vi "aft_LMS_Edit_VIs.vi"(6 "read coefficient? (F)":bool, 8 "error in":errorcluster {"code" min=0 max=0}, 9 "filter name":string, 10 "fixed-point LMS settings":T1 {"fixed-point configurations"."step size integer word length" min=0 max=0; "fixed-point configurations"."step size word length" min=0 max=0; "fixed-point configurations"."w(n) integer word length" min=0 max=0; "fixed-point configurations"."w(n) word length" min=0 max=0; "fixed-point configurations"."d(n) integer word length" min=0 max=0; "fixed-point configurations"."d(n) word length" min=0 max=0; "fixed-point configurations"."x(n) integer word length" min=0 max=0; "fixed-point configurations"."x(n) word length" min=0 max=0; "step size" min=0.0 max=0.0; "filter length" min=0 max=0}, 11 "VI ref":refnum<vi>) -> (0 "error out":errorcluster {"code" min=0 max=0})   [LabVIEW 2017, in "NI_AdaptiveFilter.lvlib"]
uses:
  <vilib>/addons/Adaptive Filters/NI_AdaptiveFilter.lvlib
  <vilib>/fxp/LVFixedPointOverflowPolicyTypeDef.ctl
  <vilib>/fxp/LVFixedPointQuantizationPolicyTypeDef.ctl
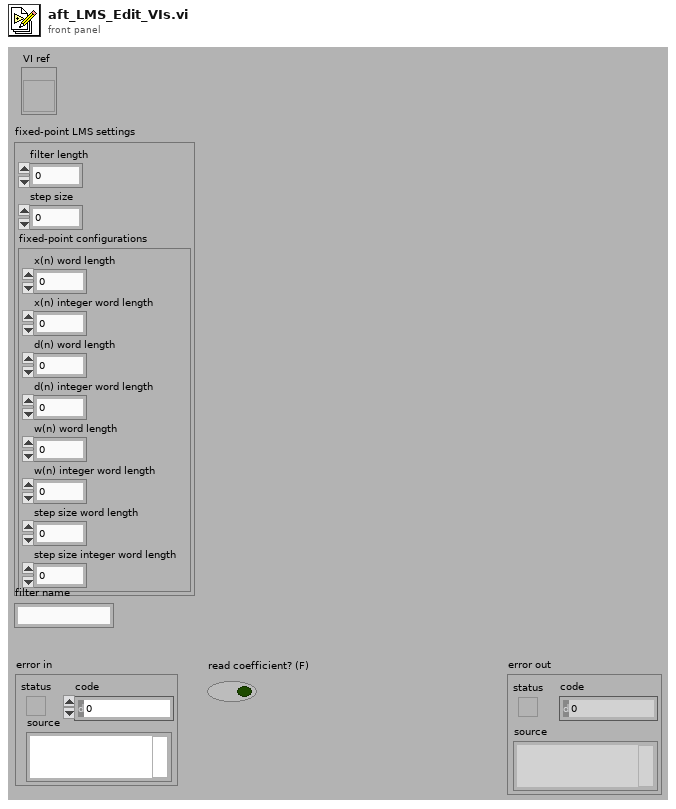
[diagram p1: front panel]
types:
  T1 = cluster{"filter length":i32, "step size":dbl, "fixed-point configurations":cluster{"x(n) word length":i32, "x(n) integer word length":i32, "d(n) word length":i32, "d(n) integer word length":i32, "w(n) word length":i32, "w(n) integer word length":i32, "step size word length":i32, "step size integer word length":i32}}
  T2 = typedef "LVFixedPointOverflowPolicyTypeDef.ctl" = enum32{"Wrap", "Saturate"}
  T3 = cluster{"x(n) word length":i32, "x(n) integer word length":i32, "d(n) word length":i32, "d(n) integer word length":i32, "w(n) word length":i32, "w(n) integer word length":i32, "step size word length":i32, "step size integer word length":i32}
  T4 = cluster{bool, u32, "x(n) integer word length":i32}
  T5 = cluster{bool, u32, "d(n) integer word length":i32}
  T6 = cluster{bool, u32, "step size integer word length":i32}
  T7 = typedef "LVFixedPointRepBitsTypeDef.ctl" = cluster{"Signed":bool, "Word Length":u32, "Integer Word Length":i32}
  T8 = typedef "LVFixedPointQuantizationPolicyTypeDef.ctl" = enum32{"Truncate", "Round-Half-Up (Asymmetric)", "Round-Half-Even"}
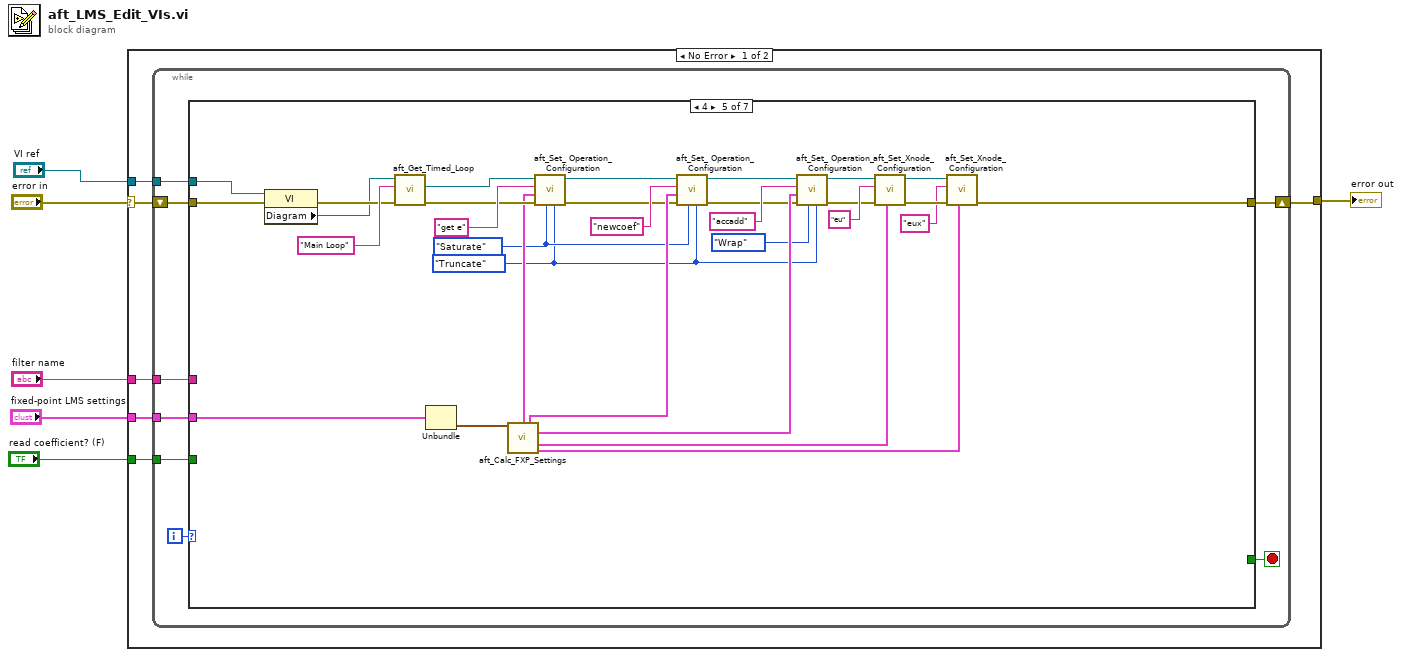
[diagram p0: block diagram]
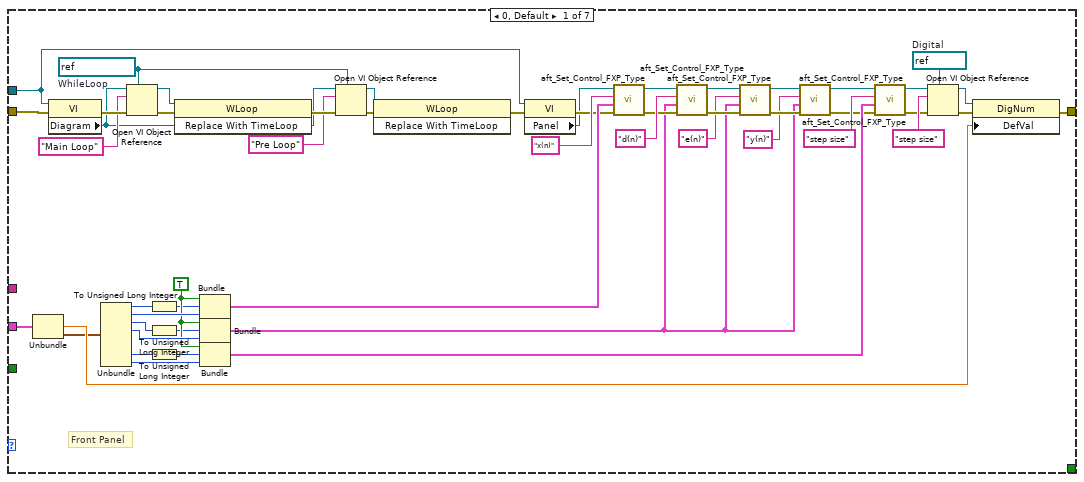
[diagram p2: hidden frame]
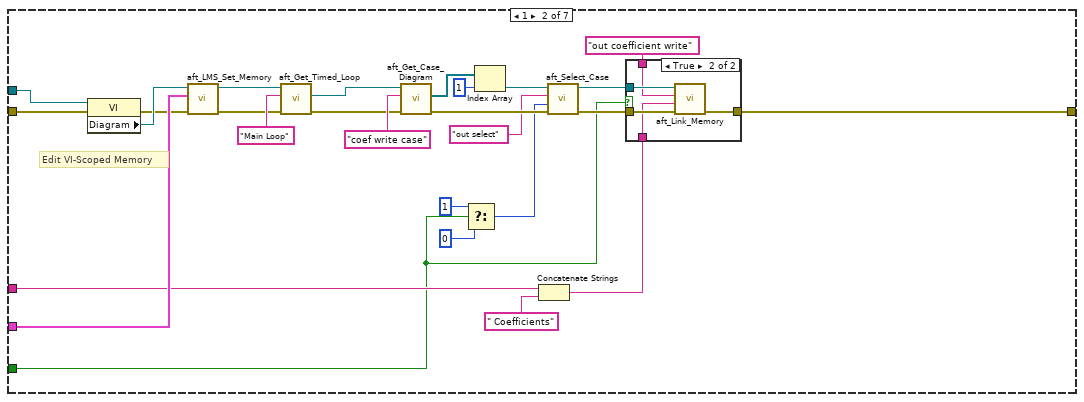
[diagram p3: hidden frame]
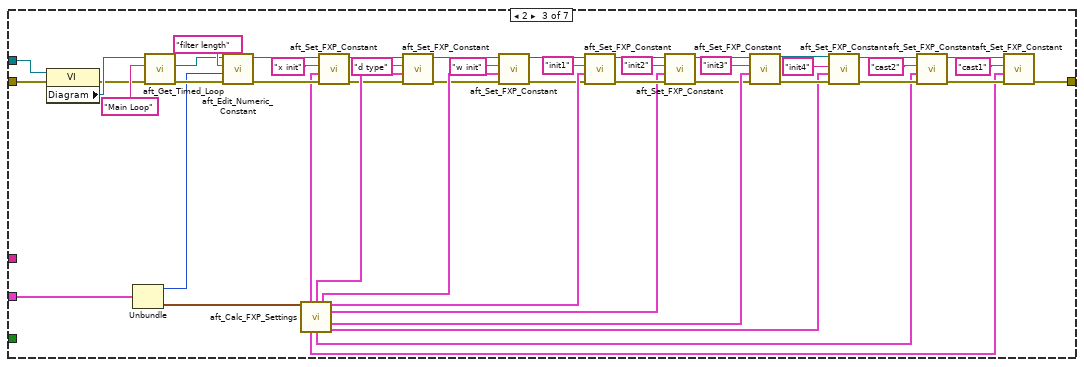
[diagram p5: hidden frame]
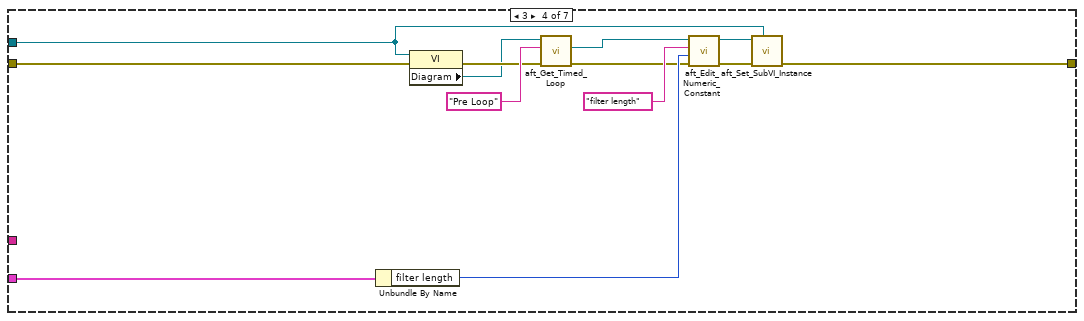
[diagram p6: hidden frame]
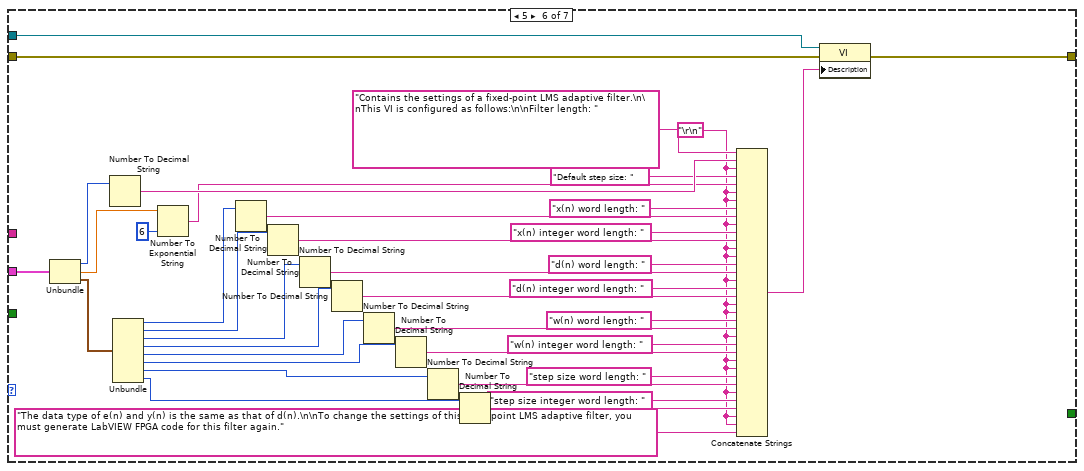
[diagram p7: hidden frame]
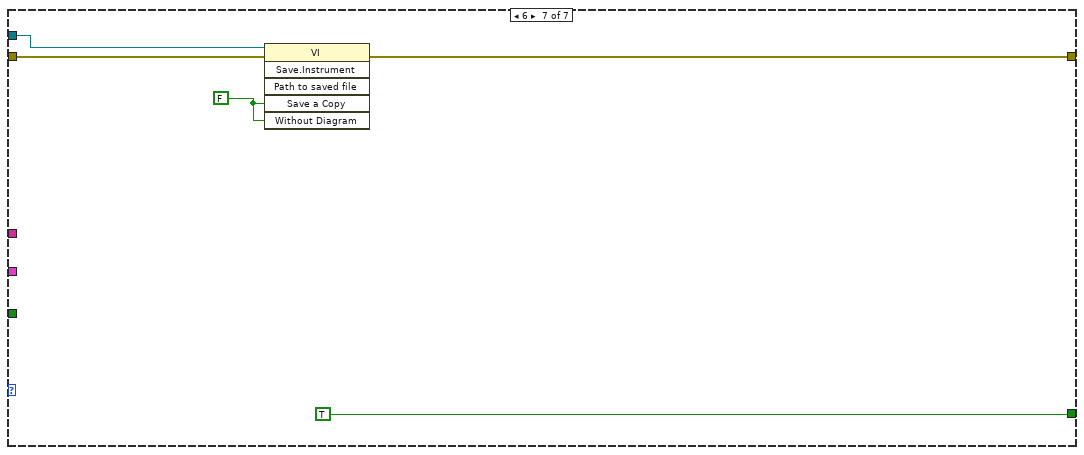
[diagram p8: hidden frame]
diagram:
  n1 = case shown="No Error" "error in" {
    selector: "error in" -> [w10 w241]
    tunnel: "VI ref" -> [w12 _]
    tunnel: [w9 w241] -> w6
    tunnel: "fixed-point LMS settings" -> [w11 _]
    tunnel: "filter name" -> [w8 _]
    tunnel: "read coefficient? (F)" -> [w7 _]
    frame No Error {
      n2 = while {
        tunnel: w12 -> [w20]
        tunnel: w11 -> [w19]
        shift-right: [w17] -> w9
        shift-left: w10 -> [w18]
        tunnel: w8 -> [w15]
        tunnel: w7 -> [w13]
        i -> [w16]
        stop <- w14 stop-if-true
        n3 = case shown="4" w16 {
          tunnel: w20 -> [w33 w94 w140 w154 w187 w197 w237]
          tunnel: w19 -> [w43 w96 w143 w161 w192 w233 _]
          tunnel: w18 -> [w34 w98 w148 w164 w196 w235 w239]
          tunnel: [w21 w78 w107 w153 w173 w234 w238] -> w17
          tunnel: w15 -> [_ w79 _ _ _ _ _]
          tunnel: [_ _ _ _ _ _ TRUE] -> w14
          tunnel: w13 -> [_ w77 _ _ _ _ _]
          frame 0, Default {
            w28 = refnum<vi> refnum  # WhileLoop
            w61 = refnum<vi> refnum  # Digital
            w58 = TRUE
            # "Front Panel"
            n4 = Unbundle(w43) -> ("step size"=w64:dbl, "fixed-point configurations"=w35:T3)  [unwired: 1 out]
            n5 = property class="VI"(reference=w33, error in=w34) -> (error out=w32:errorcluster, "Diagram"=w26:refnum<vi>)  [unwired: 1 out]
            n6 = Unbundle(w35) -> ("x(n) word length"=w66:i32, "x(n) integer word length"=w67:i32, "d(n) word length"=w68:i32, "d(n) integer word length"=w69:i32, "step size word length"=w70:i32, "step size integer word length"=w71:i32)  [unwired: 2 out]
            n7 = Open VI Object Reference(7:w28, 8:w32, 10:"Main Loop" ("name/order"), 11:w26) -> (0:w30:errorcluster, 3:w29:refnum<vi>)
            n8 = To Unsigned Long Integer(number=w66) -> (unsigned 32bit integer=w51:u32)
            n9 = To Unsigned Long Integer(number=w68) -> (unsigned 32bit integer=w52:u32)
            n10 = To Unsigned Long Integer(number=w70) -> (unsigned 32bit integer=w57:u32)
            n11 = invoke class="WLoop" method="Replace With TimeLoop"(reference=w29, error in=w30) -> (error out=w27:errorcluster)  [unwired: 1 in, 2 out]
            n12 = Bundle(w58, w51, "x(n) integer word length"=w67) -> (w47:T4)  [unwired: 1 out]
            n13 = Bundle(w58, w52, "d(n) integer word length"=w69) -> (w36:T5)  [unwired: 1 out]
            n14 = Bundle(w58, w57, "step size integer word length"=w71) -> (w59:T6)  [unwired: 1 out]
            n15 = Open VI Object Reference(7:w28, 8:w27, 10:"Pre Loop" ("name/order"), 11:w26) -> (0:w24:errorcluster, 3:w23:refnum<vi>)
            n16 = invoke class="WLoop" method="Replace With TimeLoop"(reference=w23, error in=w24) -> (error out=w22:errorcluster)  [unwired: 1 in, 2 out]
            n17 = property class="VI"(reference=w33, error in=w22) -> (error out=w45:errorcluster, "Panel"=w44:refnum<vi>)  [unwired: 1 out]
            n18 = call <vilib>:"aft_Set_Control_FXP_Type.vi"("error in (no error)"=w45, "fixed-point representation:bits"=w47, "name/order"="x(n)", "panel"=w44) -> ("error out"=w48:errorcluster, "panel out"=w49:refnum<vi>)  [unwired: 6 out]
            n19 = call <vilib>:"aft_Set_Control_FXP_Type.vi"("error in (no error)"=w48, "fixed-point representation:bits"=w36, "name/order"="d(n)", "panel"=w49) -> ("error out"=w55:errorcluster, "panel out"=w54:refnum<vi>)  [unwired: 6 out]
            n20 = call <vilib>:"aft_Set_Control_FXP_Type.vi"("error in (no error)"=w55, "fixed-point representation:bits"=w36, "name/order"="e(n)", "panel"=w54) -> ("error out"=w41:errorcluster, "panel out"=w40:refnum<vi>)  [unwired: 6 out]
            n21 = call <vilib>:"aft_Set_Control_FXP_Type.vi"("error in (no error)"=w41, "fixed-point representation:bits"=w36, "name/order"="y(n)", "panel"=w40) -> ("error out"=w38:errorcluster, "panel out"=w39:refnum<vi>)  [unwired: 6 out]
            n22 = call <vilib>:"aft_Set_Control_FXP_Type.vi"("error in (no error)"=w38, "fixed-point representation:bits"=w59, "name/order"="step size", "panel"=w39) -> ("error out"=w60:errorcluster, "panel out"=w42:refnum<vi>)  [unwired: 6 out]
            n23 = Open VI Object Reference(7:w61, 8:w60, 10:"step size" ("name/order"), 11:w42) -> (0:w63:errorcluster, 3:w62:refnum<vi>)
            n24 = property class="DigNum"(reference=w62, error in=w63, "DefVal"=w64) -> (error out=w21:errorcluster)  [unwired: 1 out]
          }
          frame 1 {
            # "Edit VI-Scoped Memory"
            n25 = property class="VI"(reference=w94, error in=w98) -> (error out=w95:errorcluster, "Diagram"=w97:refnum<vi>)  [unwired: 1 out]
            n26 = call <vilib>:"aft_LMS_Set_Memory.vi"("error in"=w95, "fixed-point LMS settings"=w96, "diagram"=w97) -> ("error out"=w75:errorcluster, "diagram out"=w73:refnum<vi>)  [unwired: 7 out]
            n27 = call <vilib>:"aft_Get_Timed_Loop.vi"("error in (no error)"=w75, "name/order"="Main Loop", "block diagram in"=w73) -> ("error out"=w74:errorcluster, "diagram out"=w72:refnum<vi>)  [unwired: 7 out]
            n28 = call <vilib>:"aft_Get_Case_Diagram.vi"("error in (no error)"=w74, "name/order"="coef write case", "Block Diagram in"=w72) -> ("error out"=w91:errorcluster, "Diagrams[]"=w93:refnum<vi>[])  [unwired: 7 out]
            n29 = Select(t=u32 1 ("visible frame"), s=w77, f=u32 0 ("visible frame")) -> (s? t:f=w86:u32)
            n30 = Index Array(array=w93, index=1) -> (element=w90:refnum<vi>)
            n31 = Concatenate Strings(w79, " Coefficients" ("string")) -> (w80:string)
            n32 = call <vilib>:"aft_Select_Case.vi"("error in (no error)"=w91, "visible frame"=w86, "name/order"="out select", "diagram in"=w90) -> ("error out"=w84:errorcluster, "diagram out"=w85:refnum<vi>)  [unwired: 6 out]
            n33 = case shown="True" w77 {
              tunnel: w85 -> [_ w104]
              tunnel: w84 -> [w99 w103]
              tunnel: "out coefficient write" ("name") -> [_ w102]
              tunnel: w80 -> [_ w101]
              tunnel: [w99 w100] -> w78
              frame False {
              }
              frame True {
                n34 = call <vilib>:"aft_Link_Memory.vi"("error in (no error)"=w103, "memory name"=w101, "name"=w102, "Diag Refnum"=w104) -> ("error out"=w100:errorcluster)  [unwired: 7 out]
              }
            }
          }
          frame 2 {
            n35 = property class="VI"(reference=w140, error in=w148) -> (error out=w146:errorcluster, "Diagram"=w147:refnum<vi>)  [unwired: 1 out]
            n36 = Unbundle(w143) -> ("filter length"=w145:i32, "fixed-point configurations"=w144:T3)  [unwired: 1 out]
            n37 = call <vilib>:"aft_Get_Timed_Loop.vi"("error in (no error)"=w146, "name/order"="Main Loop", "block diagram in"=w147) -> ("error out"=w150:errorcluster, "diagram out"=w149:refnum<vi>)  [unwired: 7 out]
            n38 = call <vilib>:"aft_Edit_Numeric_Constant.vi"("error in (no error)"=w150, "value"=w145, "name/order"="filter length", "diagram in"=w149) -> ("error out"=w137:errorcluster, "diagram out"=w139:refnum<vi>)  [unwired: 6 out]
            n39 = call <vilib>:"aft_Calc_FXP_Settings.vi"("fixed-point configurations"=w144) -> ("x"=w135:T7, "d"=w122:T7, "w"=w136:T7, "init1"=w126:T7, "init2"=w125:T7, "init3"=w124:T7, "cast 1"=w105:T7, "cast 2"=w106:T7, "init4"=w123:T7)  [unwired: 5 in, 1 out]
            n40 = call <vilib>:"aft_Set_FXP_Constant.vi"("error in (no error)"=w137, "fixed-point representation:bits"=w135, "name/order"="x init", "diagram in"=w139) -> ("error out"=w121:errorcluster, "diagram out"=w118:refnum<vi>)  [unwired: 1 in, 5 out]
            n41 = call <vilib>:"aft_Set_FXP_Constant.vi"("error in (no error)"=w121, "fixed-point representation:bits"=w122, "name/order"="d type", "diagram in"=w118) -> ("error out"=w120:errorcluster, "diagram out"=w117:refnum<vi>)  [unwired: 6 out]
            n42 = call <vilib>:"aft_Set_FXP_Constant.vi"("error in (no error)"=w120, "fixed-point representation:bits"=w136, "name/order"="w init", "diagram in"=w117) -> ("error out"=w119:errorcluster, "diagram out"=w116:refnum<vi>)  [unwired: 6 out]
            n43 = call <vilib>:"aft_Set_FXP_Constant.vi"("error in (no error)"=w119, "fixed-point representation:bits"=w126, "name/order"="init1", "diagram in"=w116) -> ("error out"=w128:errorcluster, "diagram out"=w132:refnum<vi>)  [unwired: 6 out]
            n44 = call <vilib>:"aft_Set_FXP_Constant.vi"("error in (no error)"=w128, "fixed-point representation:bits"=w125, "name/order"="init2", "diagram in"=w132) -> ("error out"=w115:errorcluster, "diagram out"=w114:refnum<vi>)  [unwired: 6 out]
            n45 = call <vilib>:"aft_Set_FXP_Constant.vi"("error in (no error)"=w115, "fixed-point representation:bits"=w124, "name/order"="init3", "diagram in"=w114) -> ("error out"=w127:errorcluster, "diagram out"=w131:refnum<vi>)  [unwired: 6 out]
            n46 = call <vilib>:"aft_Set_FXP_Constant.vi"("error in (no error)"=w127, "fixed-point representation:bits"=w123, "name/order"="init4", "diagram in"=w131) -> ("error out"=w111:errorcluster, "diagram out"=w112:refnum<vi>)  [unwired: 6 out]
            n47 = call <vilib>:"aft_Set_FXP_Constant.vi"("error in (no error)"=w111, "fixed-point representation:bits"=w106, "name/order"="cast2", "diagram in"=w112) -> ("error out"=w109:errorcluster, "diagram out"=w108:refnum<vi>)  [unwired: 6 out]
            n48 = call <vilib>:"aft_Set_FXP_Constant.vi"("error in (no error)"=w109, "fixed-point representation:bits"=w105, "name/order"="cast1", "diagram in"=w108) -> ("error out"=w107:errorcluster)  [unwired: 7 out]
          }
          frame 3 {
            n49 = Unbundle By Name(w161) -> ("filter length"=w159:i32)
            n50 = property class="VI"(reference=w154, error in=w164) -> (error out=w163:errorcluster, "Diagram"=w162:refnum<vi>)  [unwired: 1 out]
            n51 = call <vilib>:"aft_Get_Timed_Loop.vi"("error in (no error)"=w163, "name/order"="Pre Loop", "block diagram in"=w162) -> ("error out"=w155:errorcluster, "diagram out"=w156:refnum<vi>)  [unwired: 7 out]
            n52 = call <vilib>:"aft_Edit_Numeric_Constant.vi"("error in (no error)"=w155, "value"=w159, "name/order"="filter length", "diagram in"=w156) -> ("error out"=w158:errorcluster, "diagram out"=w157:refnum<vi>)  [unwired: 6 out]
            n53 = call <vilib>:"aft_Set_SubVI_Instance.vi"("VI"=w154, "error in (no error)"=w158, "diagram"=w157) -> ("error out"=w153:errorcluster)  [unwired: 8 out]
          }
          frame 4 {
            w167 = LVFixedPointQuantizationPolicyTypeDef."Truncate" ("FXP Quantization Policy")
            w168 = LVFixedPointOverflowPolicyTypeDef."Saturate" ("FXP Overflow Policy")
            n54 = property class="VI"(reference=w187, error in=w196) -> (error out=w194:errorcluster, "Diagram"=w193:refnum<vi>)  [unwired: 1 out]
            n55 = call <vilib>:"aft_Get_Timed_Loop.vi"("error in (no error)"=w194, "name/order"="Main Loop", "block diagram in"=w193) -> ("error out"=w172:errorcluster, "diagram out"=w166:refnum<vi>)  [unwired: 7 out]
            n56 = Unbundle(w192) -> ("fixed-point configurations"=w186:T3)  [unwired: 2 out]
            n57 = call <vilib>:"aft_Calc_FXP_Settings.vi"("fixed-point configurations"=w186) -> ("d"=w169:T7, "w"=w182:T7, "init2"=w178:T7, "init3"=w185:T7, "init4"=w184:T7)  [unwired: 5 in, 5 out]
            n58 = call <vilib>:"aft_Set_ Operation_Configuration.vi"("FXP Quantization Policy"=w167, "FXP Overflow Policy"=w168, "error in (no error)"=w172, "output type"=w169, "name/order"="get e", "diagram in"=w166) -> ("error out"=w171:errorcluster, "diagram out"=w170:refnum<vi>)  [unwired: 4 in]
            n59 = call <vilib>:"aft_Set_ Operation_Configuration.vi"("FXP Quantization Policy"=w167, "FXP Overflow Policy"=w168, "error in (no error)"=w171, "output type"=w182, "name/order"="newcoef", "diagram in"=w170) -> ("error out"=w175:errorcluster, "diagram out"=w174:refnum<vi>)  [unwired: 4 in]
            n60 = call <vilib>:"aft_Set_ Operation_Configuration.vi"("FXP Quantization Policy"=w167, "FXP Overflow Policy"=LVFixedPointOverflowPolicyTypeDef."Wrap", "error in (no error)"=w175, "output type"=w178, "name/order"="accadd", "diagram in"=w174) -> ("error out"=w181:errorcluster, "diagram out"=w180:refnum<vi>)  [unwired: 4 in]
            n61 = call <vilib>:"aft_Set_Xnode_Configuration.vi"("output type"=w185, "error in (no error)"=w181, "name/order"="eu", "diagram in"=w180) -> ("error out"=w189:errorcluster, "diagram out"=w190:refnum<vi>)  [unwired: 2 in, 4 out]
            n62 = call <vilib>:"aft_Set_Xnode_Configuration.vi"("output type"=w184, "error in (no error)"=w189, "name/order"="eux", "diagram in"=w190) -> ("error out"=w173:errorcluster)  [unwired: 2 in, 5 out]
          }
          frame 5 {
            w199 = "\r\n"
            n63 = Unbundle(w233) -> ("filter length"=w230:i32, "step size"=w227:dbl, "fixed-point configurations"=w232:T3)
            n64 = Number To Decimal String(number=w230) -> (decimal integer string=w229:string)  [unwired: 1 in]
            n65 = Unbundle(w232) -> ("x(n) word length"=w223:i32, "x(n) integer word length"=w220:i32, "d(n) word length"=w217:i32, "d(n) integer word length"=w213:i32, "w(n) word length"=w211:i32, "w(n) integer word length"=w210:i32, "step size word length"=w205:i32, "step size integer word length"=w203:i32)
            n66 = Number To Exponential String(number=w227, precision (6)=i16 6) -> (E-format string=w226:string)  [unwired: 2 in]
            n67 = Number To Decimal String(number=w223) -> (decimal integer string=w222:string)  [unwired: 1 in]
            n68 = Number To Decimal String(number=w220) -> (decimal integer string=w219:string)  [unwired: 1 in]
            n69 = Number To Decimal String(number=w217) -> (decimal integer string=w215:string)  [unwired: 1 in]
            n70 = Number To Decimal String(number=w213) -> (decimal integer string=w212:string)  [unwired: 1 in]
            n71 = Number To Decimal String(number=w211) -> (decimal integer string=w208:string)  [unwired: 1 in]
            n72 = Number To Decimal String(number=w210) -> (decimal integer string=w206:string)  [unwired: 1 in]
            n73 = Number To Decimal String(number=w205) -> (decimal integer string=w202:string)  [unwired: 1 in]
            n74 = Number To Decimal String(number=w203) -> (decimal integer string=w200:string)  [unwired: 1 in]
            n75 = Concatenate Strings("Contains the settings of a fixed-point LMS adaptive filter.\n\nThis VI is configured as follows:\n\nFilter length: ", w229, w199, "Default step size: " ("string"), w226, w199, w199, "x(n) word length: " ("string"), w222, w199, "x(n) integer word length: " ("string"), w219, w199, w199, "d(n) word length: " ("string"), w215, w199, "d(n) integer word length: " ("string"), w212, w199, w199, "w(n) word length: " ("string"), w208, w199, "w(n) integer word length: " ("string"), w206, w199, w199, "step size word length: " ("string"), w202, w199, "step size integer word length: " ("string"), w200, w199, w199, "The data type of e(n) and y(n) is the same as that of d(n).\n\nTo change the settings of this fixed-point LMS adaptive filter, you must generate LabVIEW FPGA code for this filter again." ("string")) -> (w218:string)
            n76 = property class="VI"(reference=w197, error in=w235, "Description"=w218) -> (error out=w234:errorcluster)  [unwired: 1 out]
          }
          frame 6 {
            w240 = FALSE ("Save a Copy")
            n77 = invoke class="VI" method="Save.Instrument"(reference=w237, error in=w239, "Save a Copy"=w240, "Without Diagram"=w240) -> (error out=w238:errorcluster)  [unwired: 2 in, 5 out]
          }
        }
      }
    }
    frame Error {
    }
  }
  "error out" <- w6
